vi "GetVMPath.vi"() -> (0 "appended path":path, 1 "filenames":string[](array[string]))   [LabVIEW 2012]
panel:
  out "sizes":i64[](array[numeric])
  out "versions":i32[](array[numeric])
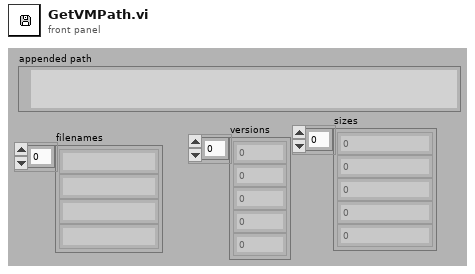
[diagram p1: front panel]
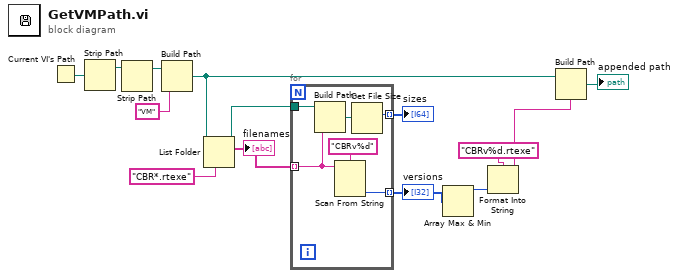
[diagram p0: block diagram]
diagram:
  n1 = Current VI's Path() -> (path=w12:path)
  n2 = Strip Path(path=w12) -> (stripped path=w11:path)  [unwired: 1 out]
  n3 = Strip Path(path=w11) -> (stripped path=w10:path)  [unwired: 1 out]
  n4 = Build Path(base path=w10, name or relative path="VM" ("path")) -> (appended path=w13:path)
  n5 = List Folder(path=w13, pattern="CBR*.rtexe") -> (path out=w2:path, filenames=w7:string[])  [unwired: 2 in, 2 out]
  "filenames" <- w7
  n6 = for {
    tunnel: w7 -> [w18] mode=indexing
    tunnel: [w19] -> w6 mode=indexing
    tunnel: w2 -> [w17]
    tunnel: [w15] -> w1 mode=indexing
    n7 = Build Path(base path=w17, name or relative path=w18) -> (appended path=w16:path)
    n8 = Scan From String(format string="CBRv%d" ("pattern"), input string=w18) -> (output 1=w19:i32)  [unwired: 3 in, 3 out]
    n9 = Get File Size(file=w16) -> (size (in bytes)=w15:i64)  [unwired: 1 in, 2 out]
  }
  "versions" <- w6
  "sizes" <- w1
  n10 = Array Max & Min(array=w6) -> (max value=w5:i32)  [unwired: 3 out]
  n11 = Format Into String(format string="CBRv%d.rtexe" ("pattern"), w5) -> (resulting string=w3:string)  [unwired: 2 in, 1 out]
  n12 = Build Path(base path=w13, name or relative path=w3) -> (appended path=→"appended path":path)
